vi "Serial_Any.vi"(8 "error in (no error)":errorcluster, 11 "Python in":cluster{"Python":refnum<k35>, "py file":path}) -> (0 "error out":errorcluster, 1 "Size":string, 2 "Size":i32, 3 "Python out":cluster{"Python":refnum<k35>, "py file":path})   [LabVIEW 2020]
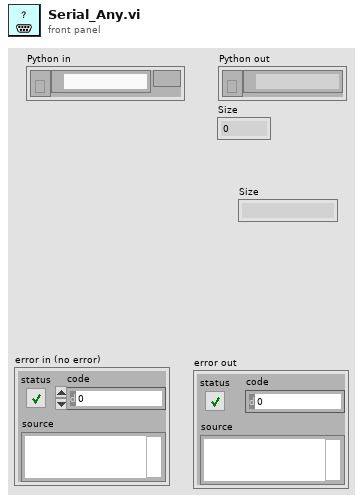
[diagram p1: front panel]
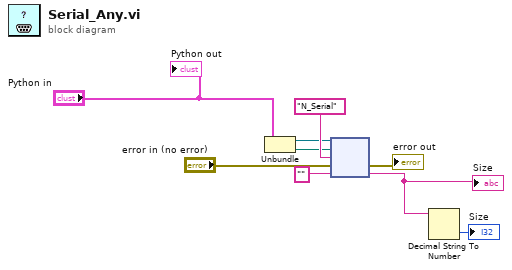
[diagram p0: block diagram]
diagram:
  n1 = Unbundle("Python in") -> ("Python"=w7:refnum<k35>, "py file"=w6:path)
  n2 = node(w7, w6, "N_Serial" ("function name"), "error in (no error)", "" ("function name")) -> (→"error out":errorcluster, w1:string)  [unwired: 3 out]
  "Size" <- w1
  n3 = Decimal String To Number(string=w1) -> (number=→"Size":i32)  [unwired: 2 in, 1 out]
  "Python out" <- "Python in"
